vi "Log Current Inc.vi"(0 "Step #":i32) -> (1 "Current & Voltage":dbl[](array[numeric]) format="%.2e", 2 "Stop":bool)   [LabVIEW 2019]
panel:
  in  "Dmm Address":refnum<visa-resource-name>
  in  "Maximum Current":dbl=0.001 min=1e-12 max=0.1 format="%.2e"
  in  "Minimum Current":dbl=1e-06 min=1e-12 max=0.1 format="%.2e"
  in  "Max Power - uW":dbl=0.005 format="%.2f"
  in  "Current Source Address":refnum<visa-resource-name>
  in  "Delay (sec)":dbl=4.0 format="%.2f"
  in  "# Steps":u32=101
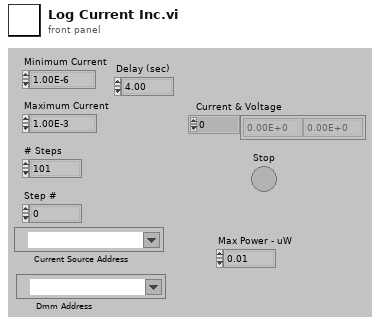
[diagram p1: front panel]
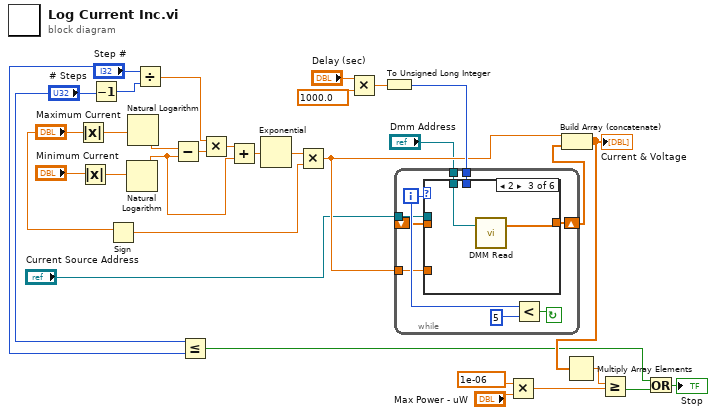
[diagram p0: block diagram]
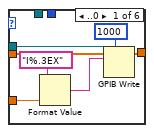
[diagram p2: hidden frame]
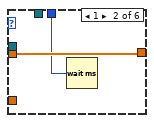
[diagram p3: hidden frame]
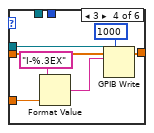
[diagram p4: hidden frame]
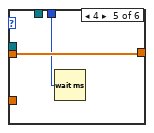
[diagram p5: hidden frame]
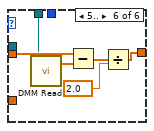
[diagram p6: hidden frame]
diagram:
  n1 = Absolute Value(x="Maximum Current") -> (abs(x)=w29:dbl)
  n2 = Absolute Value(x="Minimum Current") -> (abs(x)=w18:dbl)
  n3 = Decrement(x="# Steps") -> (x-1=w26:u32)
  n4 = Sign(1:"Maximum Current") -> (0:w20:dbl)
  n5 = Natural Logarithm(1:w18) -> (0:w17:dbl)
  n6 = Natural Logarithm(1:w29) -> (0:w28:dbl)
  n7 = Divide(x="Step #", y=w26) -> (x/y=w23:dbl)
  n8 = Subtract(x=w28, y=w17) -> (x-y=w22:dbl)
  n9 = Less Or Equal?(x="# Steps", y="Step #") -> (x <= y?=w4:bool)
  n10 = Multiply(x=w23, y=w22) -> (x*y=w24:dbl)
  n11 = Add(x=w24, y=w17) -> (x+y=w21:dbl)
  n12 = Exponential(1:w21) -> (0:w19:dbl)
  n13 = Multiply(x=w19, y=w20) -> (x*y=w11:dbl)
  n14 = Multiply(x="Delay (sec)", y=1000.0) -> (x*y=w14:dbl)
  n15 = To Unsigned Long Integer(number=w14) -> (unsigned 32bit integer=w13:u32)
  n16 = while {
    tunnel: "Dmm Address" -> [w32]
    tunnel: "Current Source Address" -> [w37]
    tunnel: w11 -> [w36]
    tunnel: w13 -> [w35]
    shift-left: _ -> [w33]
    shift-right: [w34] -> w12
    i -> [w40]
    stop <- w39 continue-if-true
    n17 = case shown="2" w40 {
      tunnel: w33 -> [w42 w48 _ w52 w58 w62]
      tunnel: [w42 w48 w49 w52 w58 w61] -> w34
      tunnel: w35 -> [_ w47 _ _ w57 _]
      tunnel: w36 -> [w44 _ _ w54 _ _]
      tunnel: w37 -> [w46 _ _ w56 _ _]
      tunnel: w32 -> [_ _ w50 _ _ w60]
      frame ..0 {
        n18 = Format Value(format string="I%.3EX", value (0)=w44) -> (output string=w41:string)  [unwired: 1 in]
        n19 = GPIB Write(0:w46, 1:w41, 4:u32 1000) -> ()  [unwired: 2 in, 2 out]
      }
      frame 1 {
        n20 = Wait (ms)(milliseconds to wait=w47) -> ()  [unwired: 1 out]
      }
      frame 2 {
        n21 = call "DMM Read.vi"("Instrument Address"=w50) -> ("Measurement"=w49:dbl[])  [unwired: 1 in, 1 out]
      }
      frame 3 {
        n22 = Format Value(format string="I-%.3EX", value (0)=w54) -> (output string=w51:string)  [unwired: 1 in]
        n23 = GPIB Write(0:w56, 1:w51, 4:u32 1000) -> ()  [unwired: 2 in, 2 out]
      }
      frame 4 {
        n24 = Wait (ms)(milliseconds to wait=w57) -> ()  [unwired: 1 out]
      }
      frame 5.. {
        n25 = call "DMM Read.vi"("Instrument Address"=w60) -> ("Measurement"=w59:dbl[])  [unwired: 1 in, 1 out]
        n26 = Subtract(x=w62, y=w59) -> (x-y=w63:dbl[])
        n27 = Divide(x=w63, y=2.0) -> (x/y=w61:dbl[])
      }
    }
    n28 = Less?(x=w40, y=5) -> (x < y?=w39:bool)
  }
  n29 = Multiply(x=1e-06, y="Max Power - uW") -> (x*y=w7:dbl)
  n30 = Build Array (concatenate)(w11, w12) -> (w8:dbl[])
  "Current & Voltage" <- w8
  n31 = Multiply Array Elements(1:w8) -> (0:w9:dbl)
  n32 = Greater Or Equal?(x=w9, y=w7) -> (x >= y?=w3:bool)
  n33 = Or(x=w4, y=w3) -> (x .or. y?=→"Stop":bool)
